vi "Get AO.vi"(0 "Module Ref":refnum<class "Modbus Master.lvclass">, 11 "error in (no error)":errorcluster) -> (4 "Modbus master out":refnum<class "Modbus Master.lvclass">, 6 "register values":u16[](array[numeric]), 15 "error out":errorcluster)   [LabVIEW 2024]
doc: "Read back analogue input status registers."
uses:
  <vilib>/NI/Modbus Library/API/Master/Modbus Master.lvclass
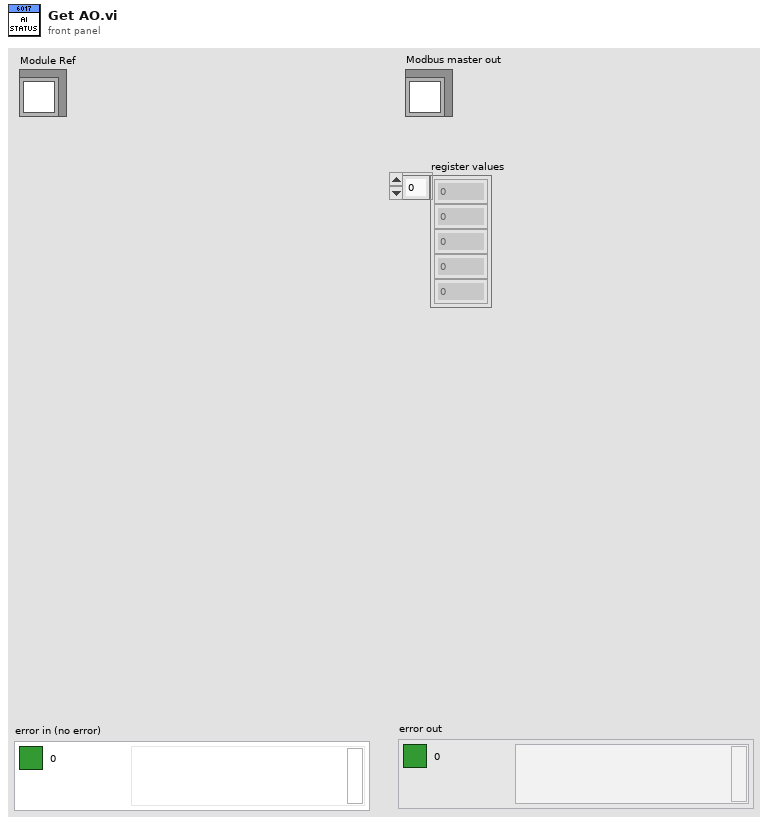
[diagram p1: front panel]
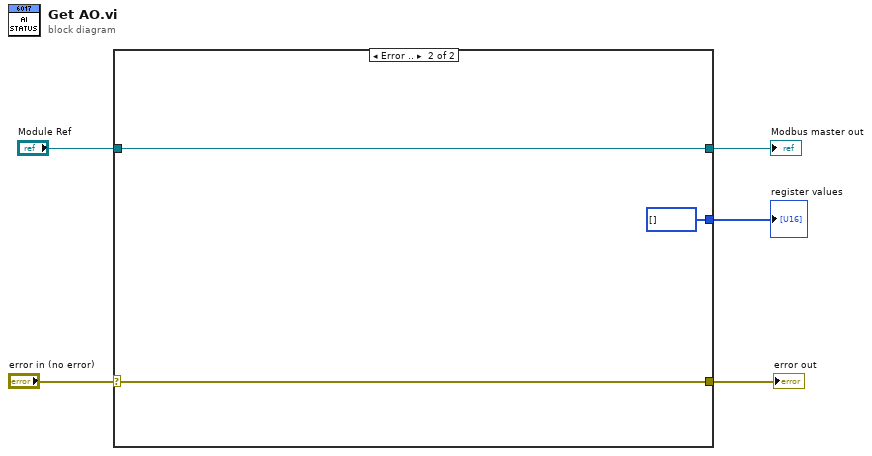
[diagram p0: block diagram]
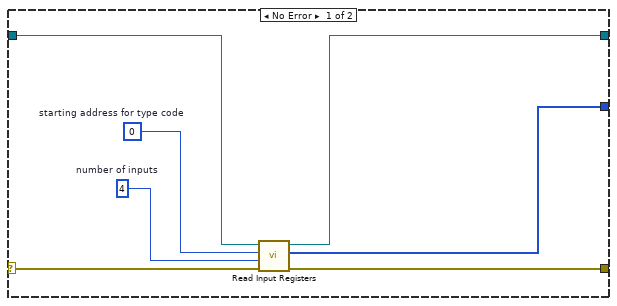
[diagram p2: hidden frame]
diagram:
  n1 = case shown="Error .." "error in (no error)" {
    selector: "error in (no error)" -> [w12 w14]
    tunnel: "Module Ref" -> [w10 w15]
    tunnel: [w7 w14] -> w3
    tunnel: [w11 w15] -> w2
    tunnel: [w6 u16[] [] ("register values")] -> w1
    frame No Error {
      w8 = u16 4  # number of inputs
      w9 = u16 0  # starting address for type code
      n2 = call-dynamic "Read Input Registers.vi"("error in"=w12, "number of inputs"=w8, "starting address"=w9, "Modbus master in"=w10) -> ("error out"=w7:errorcluster, "register values"=w6:u16[], "Modbus master out"=w11:refnum<class "Modbus Master.lvclass">)  [unwired: 5 in]
    }
    frame Error {
    }
  }
  "error out" <- w3
  "Modbus master out" <- w2
  "register values" <- w1
